vi "Host.vi"() -> ()   [LabVIEW 2018]
uses:
  <vilib>/userdefined/High Color/nirio_resource_hc.ctl
  <instrlib>/niDCPower/nidcpower.llb/niDCPower Measurement Type.ctl
  <vilib>/FPGAPlugInAG/PXI-7953R/niLvFpga_Open_PXI-7953R.vi
  <vilib>/rvi/interface/common/dynamic/niFpgaDynamicAddResources.vi
  <vilib>/FPGAPlugInAG/Dynamic/niLvFpga_Reset_Dynamic.vi
  <vilib>/FPGAPlugInAG/Dynamic/niLvFpga_Run_Dynamic.vi
  <vilib>/Utility/error.llb/Error Cluster From Error Code.vi
  <vilib>/rvi/errors/niLvFpgaAdjustHostInterfaceError.vi
  <vilib>/FPGAPlugInAG/Dynamic/niLvFpga_Close_Dynamic.vi
  <vilib>/rvi/interface/nirviOpenFPGA/nirviOpenFPGA.xnode
  FPGA Bitfiles/HCMS2975_FPGATarget_Target_JaZUenANCh4.lvbitx
  <vilib>/rvi/interface/nirviMethod/nirviMethod.xnode
  <vilib>/rvi/interface/nirviReadWriteControl/nirviReadWriteControl.xnode
  <vilib>/rvi/interface/nirviCloseFPGA/nirviCloseFPGA.xnode
  NiFpgaLv.dll
  <vilib>/rvi/interface/Simulation/niFpgaSimulationCallBeginRW.vi
panel:
  in  "RS (CR=T)":bool
  in  "CR":bool[](array[boolean])=[TRUE, TRUE, TRUE, TRUE, TRUE, TRUE, TRUE, FALSE]
  out "Картинка":bool[](array[boolean])
  in  "VLED_selcur":dbl=0.095 caption="current limit" format="%_6p"
  out "VLED":i32
  out "VLED":bool
  in  "VLED, V":dbl=5.0 caption="voltage level" format="%_6p"
  in  "VLED_curlim, A":dbl=0.1 caption="current limit" format="%_6p"
  out "VLED_cur, A":dbl caption="measurement" format="%_6g"
  out "VLED Chart":dbl(graph)=0.09491557293549348 caption="Waveform Chart 5"
  in  "V_6581":refnum<k15>="PXI1Slot2" caption="instrument handle"
  in  "Text":bool[][](array[boolean])=[[TRUE, TRUE, TRUE, TRUE, TRUE, TRUE, TRUE, TRUE, TRUE, TRUE, TRUE, FALSE, FALSE, FALSE, TRUE, TRUE, TRUE, TRUE, TRUE, FALSE, TRUE, TRUE, TRUE, TRUE, TRUE, TRUE, TRUE, TRUE, TRUE, TRUE, FALSE, FALSE, TRUE, FALSE, FALSE, FALSE, FALSE, FALSE, FALSE, FALSE], [TRUE, FALSE, FALSE, FALSE, TRUE, TRUE, FALSE, FALSE, FALSE, TRUE, TRUE, FALSE, FALSE, TRUE, TRUE, TRUE, FALSE, FALSE, FALSE, TRUE, TRUE, FALSE, FALSE, FALSE, FALSE, FALSE, FALSE, TRUE, FALSE, FALSE, FALSE, FALSE, TRUE, FALSE, FALSE, FALSE, FALSE, TRUE, FALSE, FALSE], [TRUE, FALSE, FALSE, FALSE, TRUE, TRUE, FALSE, FALSE, FALSE, TRUE, TRUE, FALSE, FALSE, TRUE, TRUE, TRUE, FALSE, FALSE, FALSE, TRUE, TRUE, FALSE, FALSE, FALSE, FALSE, FALSE, FALSE, TRUE, FALSE, FALSE, FALSE, FALSE, TRUE, FALSE, FALSE, TRUE, FALSE, FALSE, TRUE, FALSE], [TRUE, FALSE, FALSE, FALSE, TRUE, TRUE, TRUE, TRUE, TRUE, TRUE, TRUE, FALSE, TRUE, FALSE, TRUE, TRUE, TRUE, TRUE, TRUE, FALSE, TRUE, TRUE, TRUE, TRUE, TRUE, FALSE, FALSE, TRUE, FALSE, FALSE, FALSE, FALSE, TRUE, FALSE, FALSE, FALSE, FALSE, FALSE, TRUE, FALSE], [TRUE, FALSE, FALSE, FALSE, TRUE, TRUE, FALSE, FALSE, FALSE, FALSE, TRUE, TRUE, FALSE, FALSE, TRUE, TRUE, FALSE, FALSE, TRUE, FALSE, TRUE, FALSE, FALSE, FALSE, FALSE, FALSE, FALSE, TRUE, FALSE, FALSE, FALSE, FALSE, TRUE, FALSE, FALSE, FALSE, FALSE, FALSE, TRUE, FALSE], [TRUE, FALSE, FALSE, FALSE, TRUE, TRUE, FALSE, FALSE, FALSE, FALSE, TRUE, TRUE, FALSE, FALSE, TRUE, TRUE, FALSE, FALSE, FALSE, TRUE, TRUE, FALSE, FALSE, FALSE, FALSE, FALSE, FALSE, TRUE, FALSE, FALSE, FALSE, FALSE, FALSE, FALSE, FALSE, TRUE, FALSE, FALSE, TRUE, FALSE], [TRUE, FALSE, FALSE, FALSE, TRUE, TRUE, FALSE, FALSE, FALSE, FALSE, TRUE, FALSE, FALSE, FALSE, TRUE, TRUE, TRUE, TRUE, TRUE, FALSE, TRUE, TRUE, TRUE, TRUE, TRUE, FALSE, FALSE, TRUE, FALSE, FALSE, FALSE, FALSE, TRUE, FALSE, FALSE, FALSE, FALSE, TRUE, FALSE, FALSE], [FALSE, FALSE, FALSE, FALSE, FALSE, FALSE, FALSE, FALSE, FALSE, FALSE, FALSE, FALSE, FALSE, FALSE, FALSE, FALSE, FALSE, FALSE, FALSE, FALSE, FALSE, FALSE, FALSE, FALSE, FALSE, FALSE, FALSE, FALSE, FALSE, FALSE, FALSE, FALSE, FALSE, FALSE, FALSE, FALSE, FALSE, FALSE, FALSE, FALSE]]
  in  "Запись":bool
  in  "SEL_T, мс":u32=100
  in  "SIM_SEL":bool
  out "SEL":bool
  in  "VDD_selcur":dbl=0.095 caption="current limit" format="%_6p"
  out "VDD":i32
  out "VDD":bool
  in  "Период опроса, мс":u32=1000
  in  "VDD, V":dbl=5.0 caption="voltage level" format="%_6p"
  in  "VDD_curlim, A":dbl=0.1 caption="current limit" format="%_6p"
  in  "6581_curlim, A":dbl=1.0 caption="current limit" format="%_6p"
  out "VDD_cur, A":dbl caption="measurement" format="%_6g"
  out "6581_cur, A":dbl caption="measurement" format="%_6g"
  in  "6581, V":dbl=5.0 caption="voltage level" format="%_6p"
  out "6581 Chart":dbl(graph)=0.0006520018718277456
  out "VCC Chart":dbl(graph)=0.09491557293549348 caption="Waveform Chart 5"
  in  "Стоп":bool
  in  "Питание":bool
  in  "VDD_VLED":refnum<k15>="PXI1Slot2" caption="instrument handle"
  in  "resource name":T1="PXI1Slot6"
  in  "SEL":path=path "C:/VPL/LabView_PRJ/HCMS-2975_22115/LOGS"
  out "Номер образца":string="0"
  # "0"
  # "1"
  # "2"
  # "3"
  # "4"
  # "5"
  # "6"
  # "7"
  # "7"
  # "312"
  # "319"
  # "0"
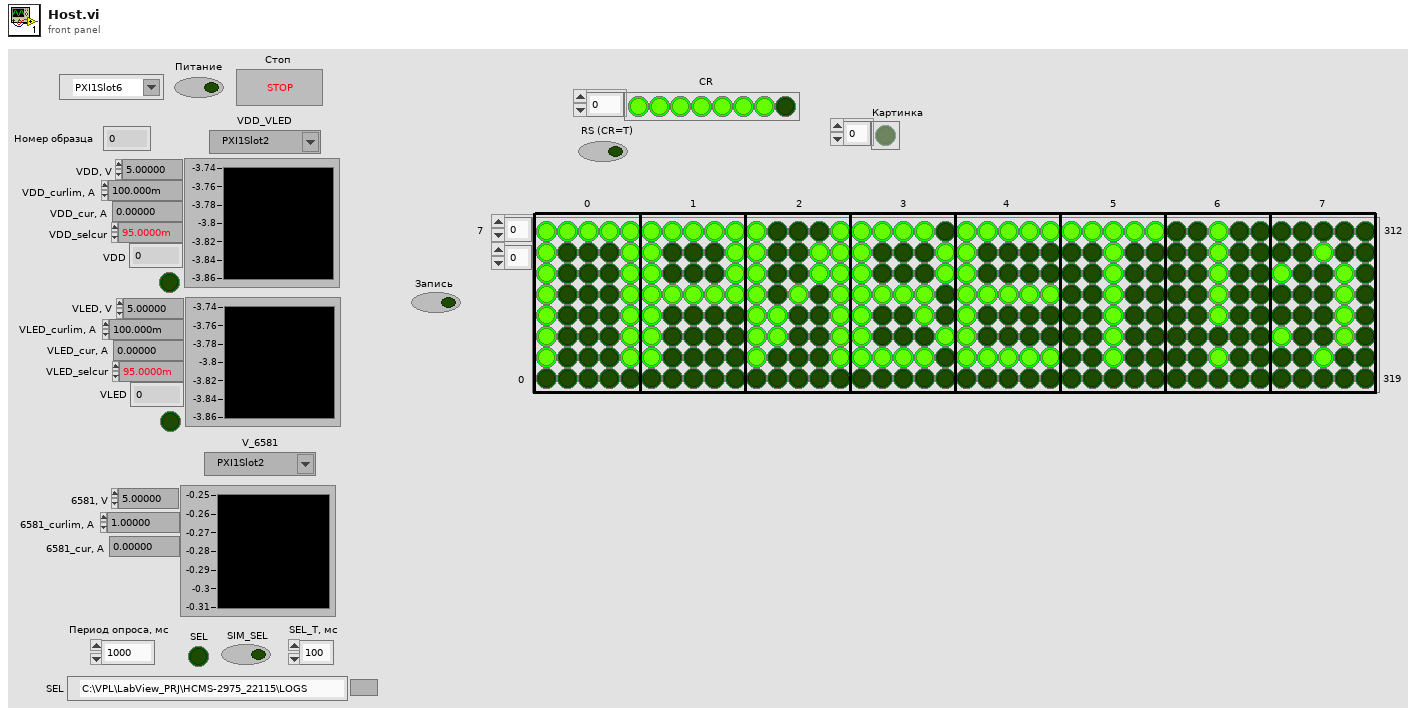
[diagram p1: front panel]
types:
  T1 = typedef "nirio_resource_hc.ctl" = tag
  T2 = enum16{"open", "replace", "create", "open or create", "replace or create", "replace or create with confirmation"}
  T3 = typedef "niDCPower Measurement Type.ctl" = i32
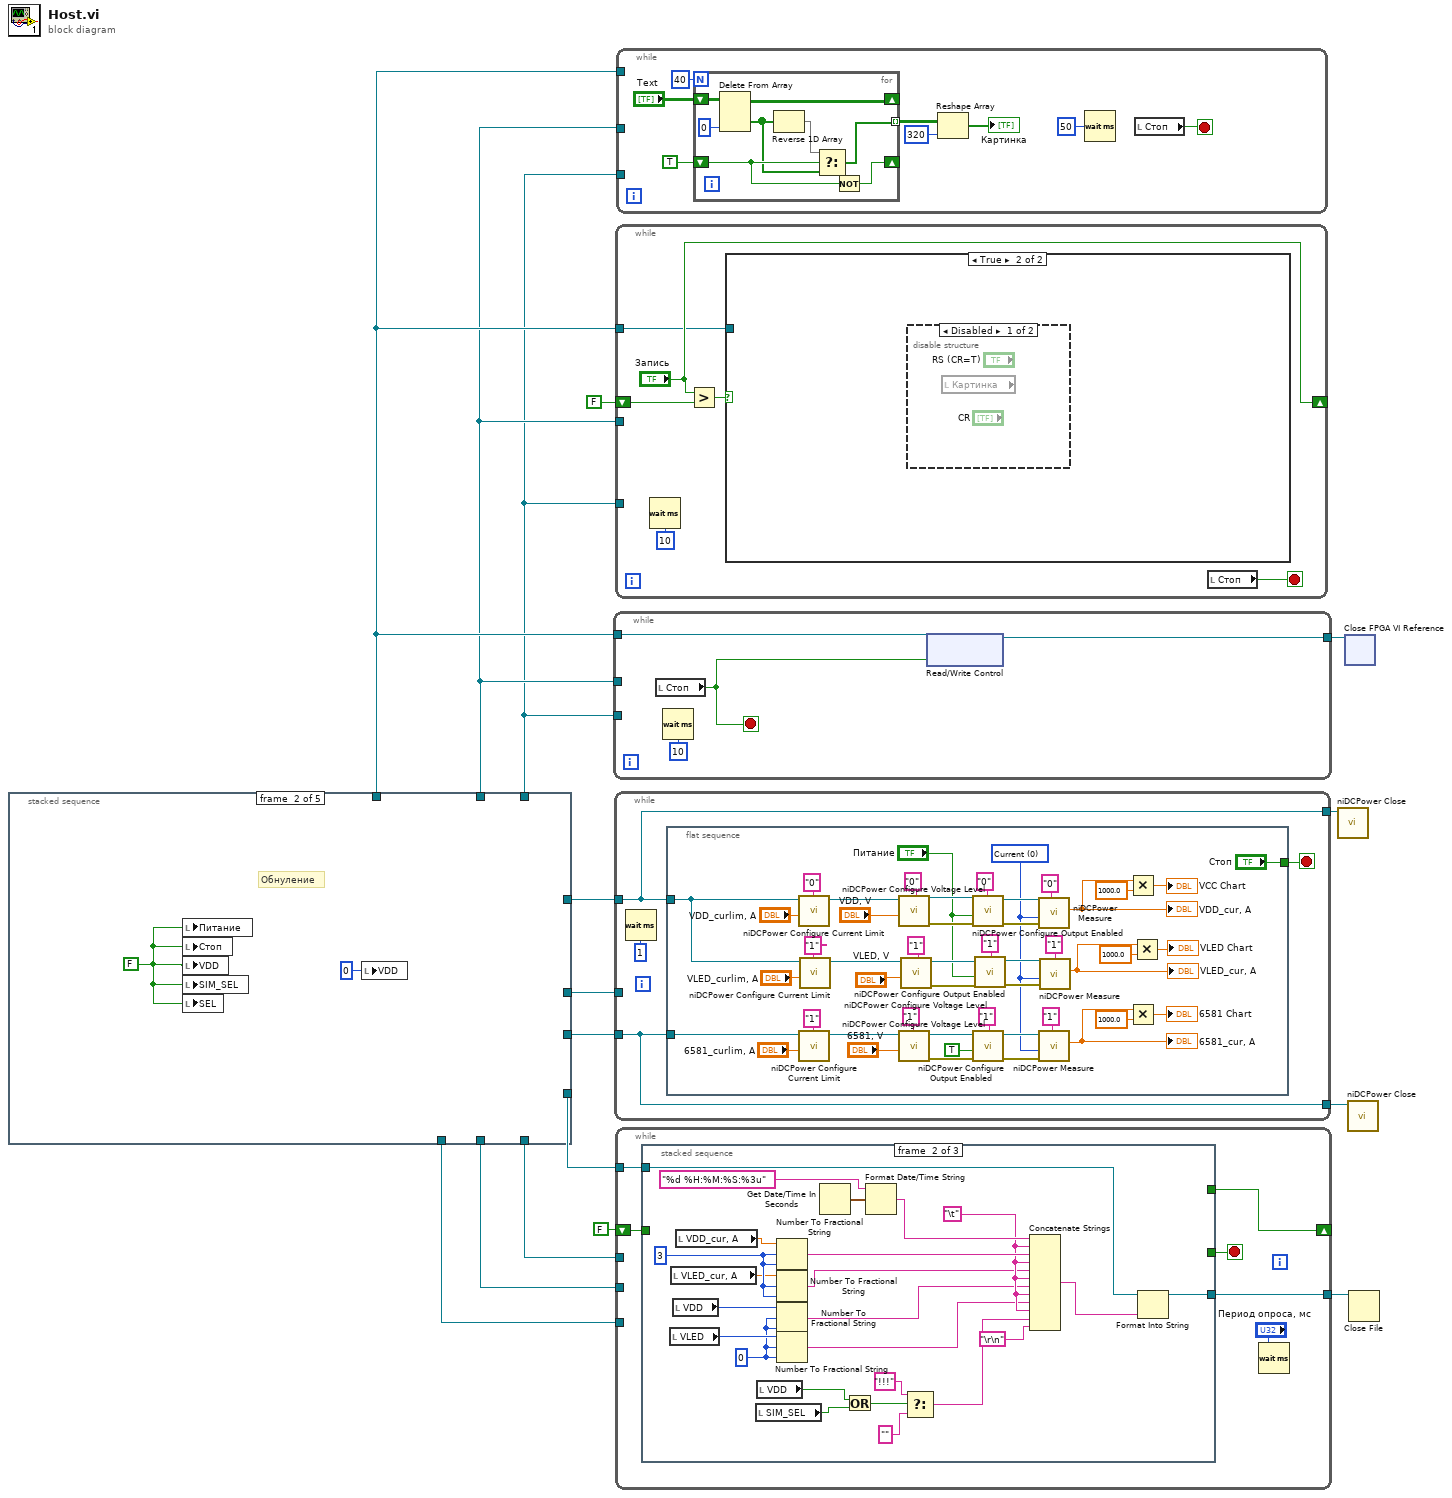
[diagram p0: block diagram]
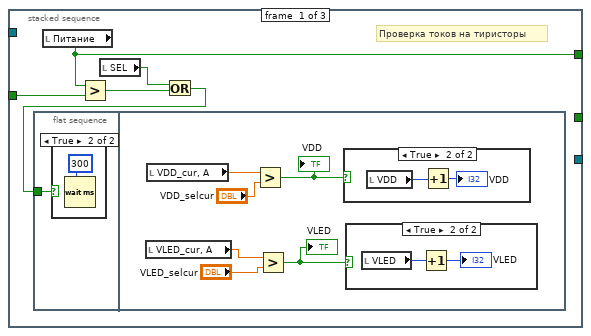
[diagram p4: hidden frame]
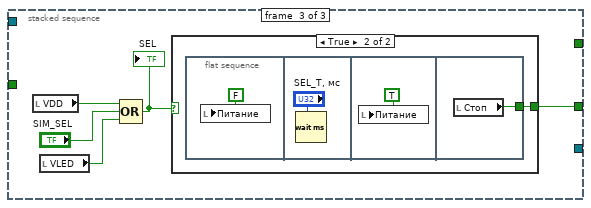
[diagram p8: hidden frame]
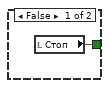
[diagram p9: hidden frame]
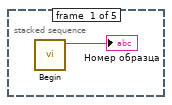
[diagram p10: hidden frame]
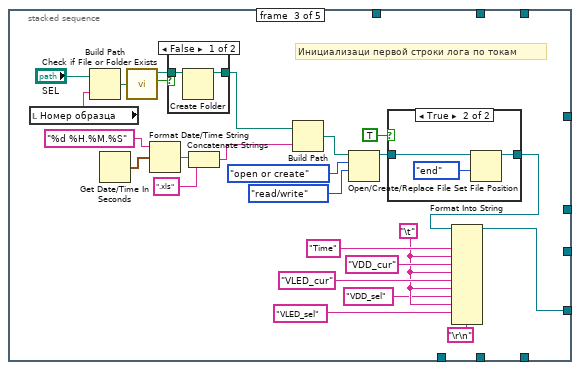
[diagram p11: hidden frame]
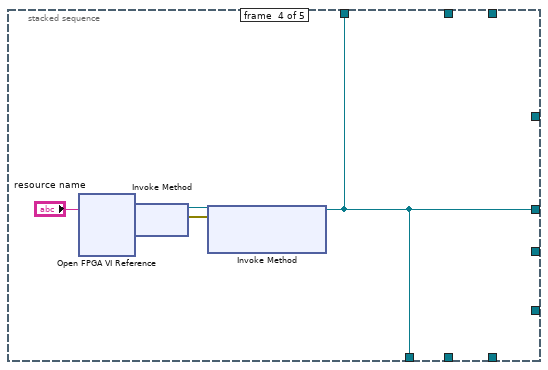
[diagram p14: hidden frame]
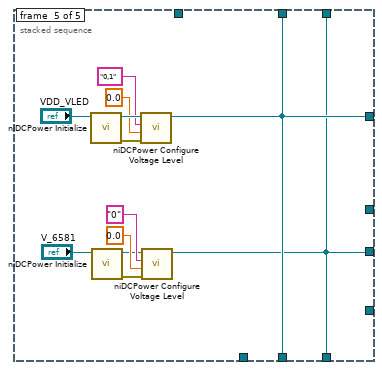
[diagram p15: hidden frame]
diagram:
  n1 = stacked-sequence {
    tunnel: [_ _ _ w52 _] -> w10
    tunnel: [_ _ w28 _ _] -> w11
    tunnel: [_ _ _ w52 _] -> w9
    tunnel: [_ _ _ w52 _] -> w3
    tunnel: [_ _ _ _ w64] -> w13
    tunnel: [_ _ _ _ w64] -> w12
    tunnel: [_ _ _ _ w64] -> w2
    tunnel: [_ _ _ _ w58] -> w6
    tunnel: [_ _ _ _ w58] -> w1
    tunnel: [_ _ _ _ w58] -> w5
    frame #0 {
      n2 = call "Begin.vi"() -> ("Номер образца 2"=→"Номер образца":string)  [unwired: 11 in]
    }
    frame #1 {
      w19 = FALSE
      # "Обнуление"
      n3 = local write "Питание"(w19) -> ()
      n4 = local write "Стоп"(w19) -> ()
      n5 = local write "VDD"(w19) -> ()
      n6 = local write "SIM_SEL"(w19) -> ()
      n7 = local write "SEL"(w19) -> ()
      n8 = local write "VDD"(0 ("VCC")) -> ()
    }
    frame #2 {
      w23 = "\t"
      # "Инициализаци первой строки лога по токам"
      n9 = local read "Номер образца"() -> (w40:string)
      n10 = Build Path(base path="SEL", name or relative path=w40) -> (appended path=w42:path)
      n11 = Get Date/Time In Seconds() -> (seconds since 1Jan1904=w35:timestamp)
      n12 = call <vilib>:"Check if File or Folder Exists.vi"("path"=w42) -> ("file or folder exists?"=w43:bool, "dup path"=w44:path)  [unwired: 8 in, 1 out]
      n13 = Format Date/Time String(time format string (%c)="%d %H.%M.%S", seconds (now)=w35) -> (date/time string=w32:string)  [unwired: 1 in]
      n14 = case shown="False" w43 {
        tunnel: w44 -> [w50 w51]
        tunnel: [w49 w51] -> w27
        frame False {
          n15 = Create Folder(path (use dialog)=w50) -> (created path=w49:path)  [unwired: 2 in, 2 out]
        }
        frame True {
        }
      }
      n16 = Concatenate Strings(w32, ".xls" ("string")) -> (w30:string)
      n17 = Build Path(base path=w27, name or relative path=w30) -> (appended path=w33:path)
      n18 = Open/Create/Replace File(file path (use dialog)=w33, operation (0:open)=T2."open or create", access (0:read/write)=enum16{"read/write", "read-only", "write-only"}."read/write") -> (refnum out=w36:refnum<file>)  [unwired: 3 in, 2 out]
      n19 = case shown="True" TRUE {
        tunnel: w36 -> [w45 w48]
        tunnel: [w45 w46] -> w29
        frame False {
        }
        frame True {
          n20 = Set File Position(refnum=w48, from (0:start)=enum16{"start", "end", "current"}."end") -> (refnum out=w46:refnum<file>)  [unwired: 2 in, 1 out]
        }
      }
      n21 = Format Into String(initial string=w29, "Time" ("input 1"), w23, "VDD_cur" ("input 1"), w23, "VLED_cur" ("input 1"), w23, "VDD_sel" ("input 1"), w23, "VLED_sel" ("input 1"), "\r\n") -> (resulting string=w28:refnum<file>)  [unwired: 2 in, 1 out]
    }
    frame #3 {
      n22 = xnode "Open FPGA VI Reference"("resource name"="resource name") -> ("FPGA VI Reference Out"=w57:refnum<k20>, "error out"=w55:errorcluster)  [unwired: 1 in]
      n23 = xnode "Invoke Method"("FPGA VI Reference In"=w57, "error in"=w55) -> ("FPGA VI Reference Out"=w54:refnum<k20>, "error out"=w56:errorcluster)
      n24 = xnode "Invoke Method"("FPGA VI Reference In"=w54, "error in"=w56) -> ("FPGA VI Reference Out"=w52:refnum<k20>)  [unwired: 1 in, 1 out]
    }
    frame #4 {
      n25 = call <instrlib>:"niDCPower Initialize.vi"("resource name"="VDD_VLED") -> ("error out"=w68:errorcluster, "instrument handle out"=w69:refnum<k15>)  [unwired: 3 in, 6 out]
      n26 = call <instrlib>:"niDCPower Initialize.vi"("resource name"="V_6581") -> ("error out"=w60:errorcluster, "instrument handle out"=w59:refnum<k15>)  [unwired: 3 in, 6 out]
      n27 = call <instrlib>:"niDCPower Configure Voltage Level.vi"("error in (no error)"=w68, "voltage level"=0.0, "channel name"="0,1", "instrument handle"=w69) -> ("instrument handle out"=w64:refnum<k15>)  [unwired: 6 in, 1 out]
      n28 = call <instrlib>:"niDCPower Configure Voltage Level.vi"("error in (no error)"=w60, "voltage level"=0.0, "channel name"="0", "instrument handle"=w59) -> ("instrument handle out"=w58:refnum<k15>)  [unwired: 6 in, 1 out]
    }
  }
  n29 = while {
    tunnel: w3 -> [w72]
    tunnel: w2 -> [_]
    tunnel: [w70] -> w8
    tunnel: w1 -> [_]
    stop <- w71 stop-if-true
    n30 = local read "Стоп"() -> (w71:bool)
    n31 = Wait (ms)(milliseconds to wait=u32 10) -> ()  [unwired: 1 out]
    n32 = xnode "Read/Write Control"("FPGA VI Reference In"=w72, "Stop_FPGA"=w71) -> ("FPGA VI Reference Out"=w70:refnum<k20>)  [unwired: 1 in, 1 out]
  }
  n33 = while {
    tunnel: w13 -> [w75]
    tunnel: [w75] -> w14
    tunnel: w10 -> [_]
    tunnel: w6 -> [w74]
    tunnel: [w74] -> w4
    stop <- w76 stop-if-true
    n34 = Wait (ms)(milliseconds to wait=u32 1) -> ()  [unwired: 1 out]
    n35 = flat-sequence {
      tunnel: w75 -> [w94]
      tunnel: ["Стоп"] -> w76
      tunnel: w74 -> [w95]
      frame #0 {
        w78 = T3 0 items=["Current", "Voltage"] ("measurement type")
        n36 = call <instrlib>:"niDCPower Configure Current Limit.vi"("current limit"="VDD_curlim, A", "channel name"="0", "instrument handle"=w94) -> ("instrument handle out"=w115:refnum<k15>)  [unwired: 7 in, 1 out]
        n37 = call <instrlib>:"niDCPower Configure Current Limit.vi"("current limit"="6581_curlim, A", "channel name"="1", "instrument handle"=w95) -> ("instrument handle out"=w116:refnum<k15>)  [unwired: 7 in, 1 out]
        n38 = call <instrlib>:"niDCPower Configure Current Limit.vi"("current limit"="VLED_curlim, A", "channel name"="1", "instrument handle"=w94) -> ("instrument handle out"=w91:refnum<k15>)  [unwired: 7 in, 1 out]
        n39 = call <instrlib>:"niDCPower Configure Voltage Level.vi"("voltage level"="VDD, V", "channel name"="0", "instrument handle"=w115) -> ("error out"=w108:errorcluster, "instrument handle out"=w111:refnum<k15>)  [unwired: 7 in]
        n40 = call <instrlib>:"niDCPower Configure Voltage Level.vi"("voltage level"="6581, V", "channel name"="1", "instrument handle"=w116) -> ("error out"=w109:errorcluster, "instrument handle out"=w110:refnum<k15>)  [unwired: 7 in]
        n41 = call <instrlib>:"niDCPower Configure Voltage Level.vi"("voltage level"="VLED, V", "channel name"="1", "instrument handle"=w91) -> ("error out"=w80:errorcluster, "instrument handle out"=w90:refnum<k15>)  [unwired: 7 in]
        n42 = call <instrlib>:"niDCPower Configure Output Enabled.vi"("error in (no error)"=w108, "output enabled"="Питание", "channel name"="0", "instrument handle"=w111) -> ("error out"=w120:errorcluster, "instrument handle out"=w119:refnum<k15>)  [unwired: 6 in]
        n43 = call <instrlib>:"niDCPower Configure Output Enabled.vi"("error in (no error)"=w109, "output enabled"=TRUE, "channel name"="1", "instrument handle"=w110) -> ("error out"=w121:errorcluster, "instrument handle out"=w122:refnum<k15>)  [unwired: 6 in]
        n44 = call <instrlib>:"niDCPower Configure Output Enabled.vi"("error in (no error)"=w80, "output enabled"="Питание", "channel name"="1", "instrument handle"=w90) -> ("error out"=w79:errorcluster, "instrument handle out"=w89:refnum<k15>)  [unwired: 6 in]
        n45 = call <instrlib>:"niDCPower Measure.vi"("error in (no error)"=w120, "measurement type"=w78, "channel name"="0", "instrument handle"=w119) -> ("measurement"=w101:dbl)  [unwired: 5 in, 2 out]
        "VDD_cur, A" <- w101
        n46 = call <instrlib>:"niDCPower Measure.vi"("error in (no error)"=w121, "measurement type"=w78, "channel name"="1", "instrument handle"=w122) -> ("measurement"=w102:dbl)  [unwired: 5 in, 2 out]
        "6581_cur, A" <- w102
        n47 = call <instrlib>:"niDCPower Measure.vi"("error in (no error)"=w79, "measurement type"=w78, "channel name"="1", "instrument handle"=w89) -> ("measurement"=w82:dbl)  [unwired: 5 in, 2 out]
        "VLED_cur, A" <- w82
        n48 = Multiply(x=w101, y=1000.0) -> (x*y=→"VCC Chart":dbl)
        n49 = Multiply(x=w102, y=1000.0) -> (x*y=→"6581 Chart":dbl)
        n50 = Multiply(x=w82, y=1000.0) -> (x*y=→"VLED Chart":dbl)
      }
    }
  }
  n51 = while {
    tunnel: w3 -> [w127]
    tunnel: w2 -> [_]
    shift-right: ["Запись"] -> _
    shift-left: FALSE ("Сообщение") -> [w131]
    tunnel: w1 -> [_]
    stop <- w129 stop-if-true
    n52 = Wait (ms)(milliseconds to wait=u32 10) -> ()  [unwired: 1 out]
    n53 = Greater?(x="Запись", y=w131) -> (0:w128:bool)
    n54 = case shown="True" w128 {
      tunnel: w127 -> [_ _]
      frame False {
      }
      frame True {
        n55 = disable-structure shown="Disabled" {
          frame Disabled {
            n56 = local read "Картинка"() -> ()  [unwired: 1 out]
          }
          frame Enabled {
          }
        }
      }
    }
    n57 = local read "Стоп"() -> (w129:bool)
  }
  n58 = while {
    shift-right: [w137] -> _
    shift-left: FALSE -> [w136]
    tunnel: w11 -> [w135]
    tunnel: [w133] -> w15
    tunnel: w12 -> [_]
    tunnel: w9 -> [_]
    tunnel: w5 -> [_]
    stop <- w134 stop-if-true
    n59 = stacked-sequence {
      tunnel: [w141 _ _] -> w137
      tunnel: w136 -> [w142 _ _]
      tunnel: w135 -> [_ w171 _]
      tunnel: [_ _ w181] -> w134
      tunnel: [_ w169 _] -> w133
      frame #0 {
        # "Проверка токов на тиристоры"
        n60 = flat-sequence {
          tunnel: w138 -> [w143]
          frame #0 {
            n61 = case shown="True" w143 {
              frame False {
              }
              frame True {
                n62 = Wait (ms)(milliseconds to wait=u32 300) -> ()  [unwired: 1 out]
              }
            }
          }
          frame #1 {
            n63 = local read "VLED_cur, A"() -> (w147:dbl)
            n64 = local read "VDD_cur, A"() -> (w148:dbl)
            n65 = Greater?(x=w148, y="VDD_selcur") -> (0:w149:bool)
            "VDD" <- w149
            n66 = Greater?(x=w147, y="VLED_selcur") -> (0:w145:bool)
            "VLED" <- w145
            n67 = case shown="True" w149 {
              frame False {
              }
              frame True {
                n68 = local read "VDD"() -> (w154:i32)
                n69 = Increment(x=w154) -> (x+1=→"VDD":i32)
              }
            }
            n70 = case shown="True" w145 {
              frame False {
              }
              frame True {
                n71 = local read "VLED"() -> (w152:i32)
                n72 = Increment(x=w152) -> (x+1=→"VLED":i32)
              }
            }
          }
        }
        n73 = local read "Питание"() -> (w141:bool)
        n74 = Greater?(x=w141, y=w142) -> (0:w140:bool)
        n75 = local read "SEL"() -> (w139:bool)
        n76 = Or(x=w139, y=w140) -> (x .or. y?=w138:bool)
      }
      frame #1 {
        w160 = i16 0 ("width (-)")
        w164 = i16 3 ("width (-)")
        w165 = "\t"
        n77 = local read "VLED"() -> (w161:i32)
        n78 = local read "VLED_cur, A"() -> (w163:dbl)
        n79 = local read "VDD"() -> (w162:i32)
        n80 = local read "VDD_cur, A"() -> (w170:dbl)
        n81 = local read "SIM_SEL"() -> (w168:bool)
        n82 = local read "VDD"() -> (w167:bool)
        n83 = Number To Fractional String(number=w170, width (-)=w164, precision (6)=w164) -> (F-format string=w172:string)  [unwired: 1 in]
        n84 = Number To Fractional String(number=w163, width (-)=w164, precision (6)=w164) -> (F-format string=w159:string)  [unwired: 1 in]
        n85 = Number To Fractional String(number=w162, width (-)=w160, precision (6)=w160) -> (F-format string=w158:string)  [unwired: 1 in]
        n86 = Number To Fractional String(number=w161, width (-)=w160, precision (6)=w160) -> (F-format string=w157:string)  [unwired: 1 in]
        n87 = Get Date/Time In Seconds() -> (seconds since 1Jan1904=w178:timestamp)
        n88 = Or(x=w167, y=w168) -> (x .or. y?=w166:bool)
        n89 = Format Date/Time String(time format string (%c)="%d %H:%M:%S:%3u", seconds (now)=w178) -> (date/time string=w173:string)  [unwired: 1 in]
        n90 = Select(t="!!!", s=w166, f="") -> (s? t:f=w156:string)
        n91 = Concatenate Strings(w173, w165, w172, w165, w159, w165, w158, w165, w157, w165, w156, "\r\n") -> (w177:string)
        n92 = Format Into String(initial string=w171, w177) -> (resulting string=w169:refnum<file>)  [unwired: 2 in, 1 out]
      }
      frame #2 {
        n93 = local read "VDD"() -> (w183:bool)
        n94 = local read "VLED"() -> (w179:bool)
        n95 = Compound Arithmetic op=OR(w183, "SIM_SEL", w179) -> (w182:bool)
        "SEL" <- w182
        n96 = case shown="True" w182 {
          tunnel: [w184 w185] -> w181
          frame False {
            n97 = local read "Стоп"() -> (w184:bool)
          }
          frame True {
            n98 = flat-sequence {
              tunnel: [w189] -> w185
              frame #0 {
                n99 = local write "Питание"(FALSE ("SYS_RESET")) -> ()
              }
              frame #1 {
                n100 = Wait (ms)(milliseconds to wait="SEL_T, мс") -> ()  [unwired: 1 out]
              }
              frame #2 {
                n101 = local write "Питание"(TRUE ("SYS_RESET")) -> ()
              }
              frame #3 {
                n102 = local read "Стоп"() -> (w189:bool)
              }
            }
          }
        }
      }
    }
    n103 = Wait (ms)(milliseconds to wait="Период опроса, мс") -> ()  [unwired: 1 out]
  }
  n104 = while {
    tunnel: w3 -> [_]
    tunnel: w2 -> [_]
    tunnel: w1 -> [_]
    stop <- w197 stop-if-true
    n105 = for {
      N: 40 -> [_]
      shift-right: [w204] -> _
      shift-left: "Text" -> [w205]
      tunnel: [w203] -> w196 mode=indexing
      shift-right: [w200] -> _
      shift-left: TRUE -> [w201]
      n106 = Delete From Array(array=w205, index (col)=0 ("disabled index (col)")) -> (deleted portion=w199:bool[], array with subset deleted=w204:bool[][])  [unwired: 2 in]
      n107 = Reverse 1D Array(array=w199) -> (reversed array=w198:bool[])
      n108 = Select(t=w198, s=w201, f=w199) -> (s? t:f=w203:bool[])
      n109 = Not(x=w201) -> (.not. x?=w200:bool)
    }
    n110 = Reshape Array(w196, 320 ("dimension size")) -> (→"Картинка":bool[])
    n111 = Wait (ms)(milliseconds to wait=u32 50) -> ()  [unwired: 1 out]
    n112 = local read "Стоп"() -> (w197:bool)
  }
  n113 = call <instrlib>:"niDCPower Close.vi"("instrument handle"=w14) -> ()  [unwired: 10 in, 1 out]
  n114 = xnode "Close FPGA VI Reference"("FPGA VI Reference In"=w8) -> ()  [unwired: 1 in, 1 out]
  n115 = call <instrlib>:"niDCPower Close.vi"("instrument handle"=w4) -> ()  [unwired: 10 in, 1 out]
  n116 = Close File(refnum=w15) -> ()  [unwired: 1 in, 2 out]
